vi "value2range_VAC.vi"(2 "Voltage [V]":dbl) -> (1 "Limited voltage [V]":dbl, 4 "Positive or zero":bool, 6 "Range limit [V]":dbl, 7 "Range [-]":i32, 8 "Positive":bool, 9 "Overflow":bool)   [LabVIEW 2020, in "Datron D4xxx.lvlib"]
doc: "This VI converts input voltage value to range code. It is usefull for \"manual autorange\"."
uses:
  Datron D4xxx.lvlib
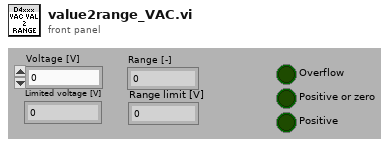
[diagram p1: front panel]
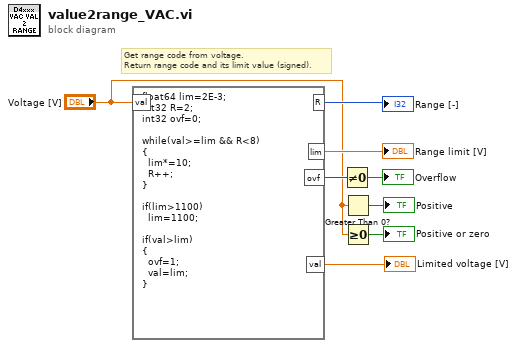
[diagram p0: block diagram]
diagram:
  # "Get range code from voltage.\nReturn range code and its limit value (signed)."
  n1 = formula code="float64 lim=2E-3;\nint32 R=2;\nint32 ovf=0;\n\nwhile(val>=lim && R<8)\n{\n  lim*=10;\n  R++;\n}\n\nif(lim>1100)\n  lim=1100;\n\nif(val>lim)\n{\n  ovf=1;\n  val=lim;\n}"("val"="Voltage [V]") -> ("R"=→"Range [-]":i32, "lim"=→"Range limit [V]":dbl, "ovf"=w6:i32, "val"=→"Limited voltage [V]":dbl)
  n2 = Not Equal To 0?(x=w6) -> (x != 0?=→"Overflow":bool)
  n3 = Greater Than 0?(x="Voltage [V]") -> (x > 0?=→"Positive":bool)
  n4 = Greater Or Equal To 0?(x="Voltage [V]") -> (x >= 0?=→"Positive or zero":bool)
